vi "Main.vi"() -> ()   [LabVIEW 2018]
uses:
  Banda--control.ctl
  Banda Tolerancia--control.ctl
  states--control.ctl
  data--control.ctl
panel:
  out "in E12?":bool caption="Cumple E12?"
  out "in E24?":bool caption="Cumple E24?"
  in  "Tol":T1 caption="Tolerancia"
  out "Tol":u32(colorbox)
  out "3b":u32(colorbox)
  out "2b":u32(colorbox)
  out "1b":u32(colorbox)
  in  "stop":bool
  in  "3° banda":T2
  in  "2° banda":T2
  in  "1° banda":T2
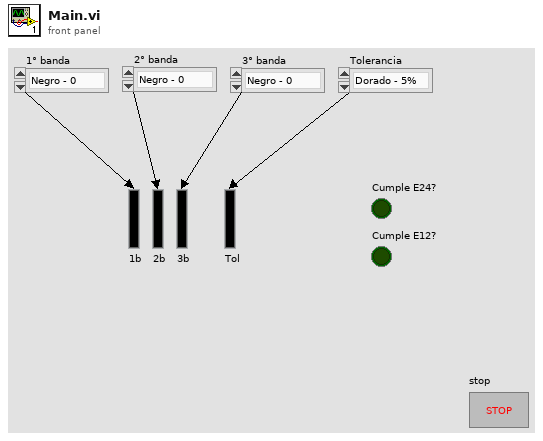
[diagram p1: front panel]
types:
  T1 = typedef "Banda Tolerancia--control.ctl" = enum16{"Dorado - 5%", "Plata - 10%"}
  T2 = typedef "Banda--control.ctl" = enum16{"Negro - 0", "Marrón - 1", "Rojo - 2", "Naranja - 3", "Amarillo - 4", "Verde - 5", "Azul - 6", "Violeta - 7", "Gris - 8", "Blanco - 9"}
  T3 = typedef "data--control.ctl" = cluster{"Number":i32, "Sting":string, "Boolean":bool, "1b Refn":refnum<vi>, "2b Refn":refnum<vi>, "3b Refn":refnum<vi>, "Tol Refn":refnum<vi>, "E24 Series":u8[], "E12 Series":u8[], "in E24?":bool, "in E12?":bool, "1° banda":T2, "2° banda":T2, "3° banda":T2, "Tolerancia":T1, "band 1":u32, "band 2":u32, "band 3":u32, "Tol":u32}
  T4 = typedef "states--control.ctl" = enum16{"Initialize", "Read E24 Series", "Read E12 Series", "Initialize Colors", "Wait", "Set Resistance Colors", "Verify E12 Series", "Verify E24 Series ", "Set Tol", "Error", "Shutdown"}
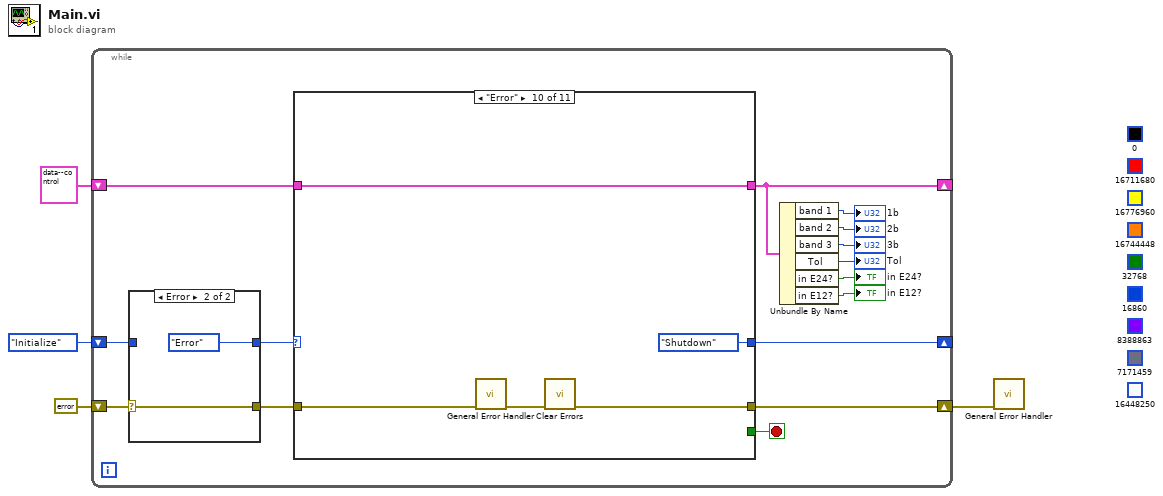
[diagram p0: block diagram]
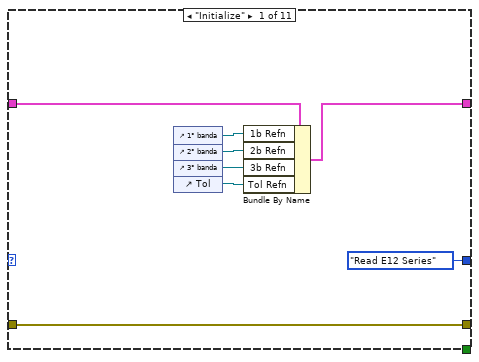
[diagram p3: hidden frame]
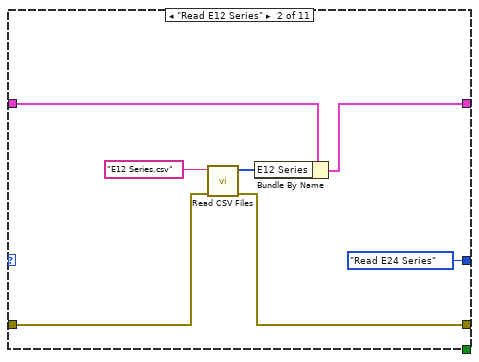
[diagram p4: hidden frame]
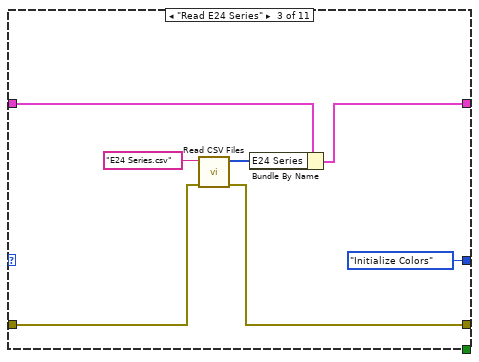
[diagram p5: hidden frame]
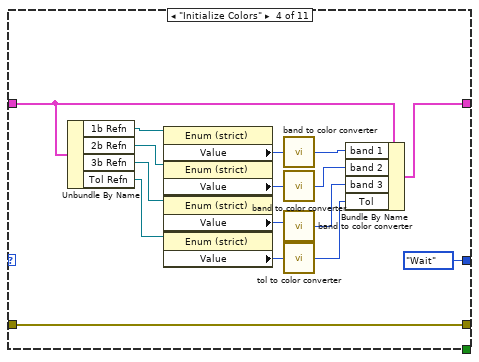
[diagram p6: hidden frame]
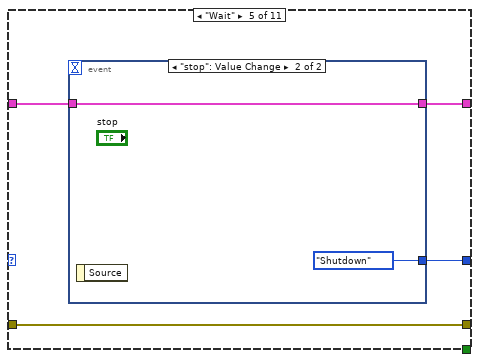
[diagram p7: hidden frame]
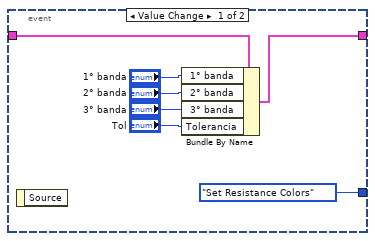
[diagram p8: hidden frame]
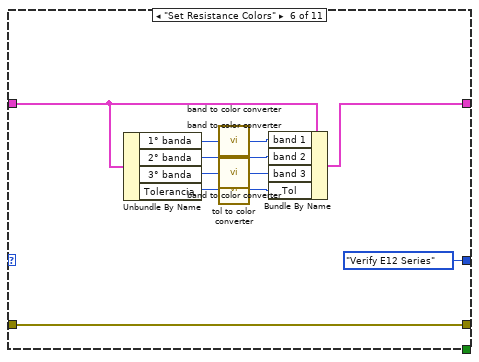
[diagram p9: hidden frame]
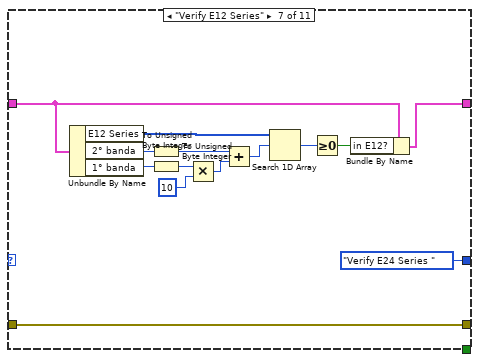
[diagram p10: hidden frame]
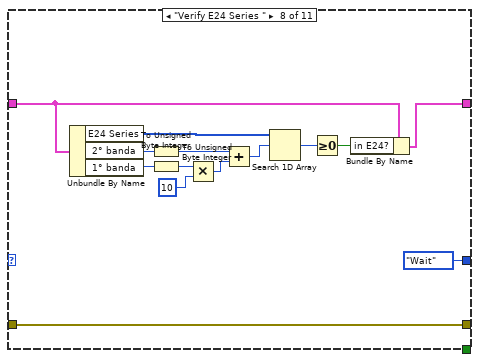
[diagram p11: hidden frame]
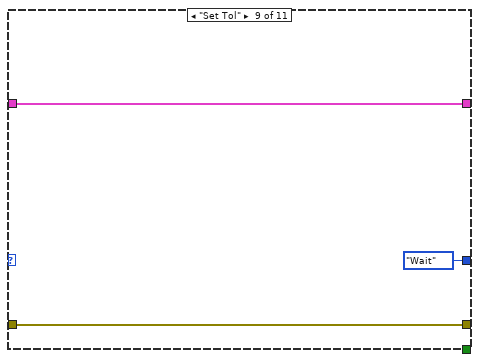
[diagram p12: hidden frame]
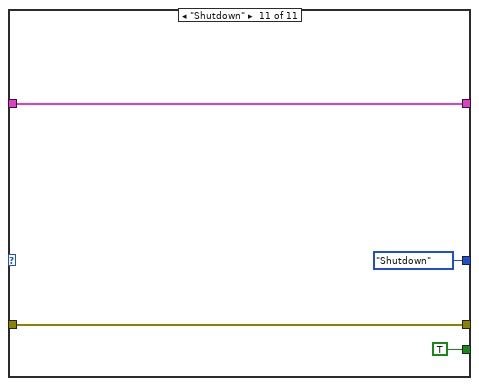
[diagram p13: hidden frame]
diagram:
  (unwired) u32 16448250
  (unwired) u32 7171459
  (unwired) u32 8388863
  (unwired) u32 16860
  (unwired) u32 32768
  (unwired) u32 16744448
  (unwired) u32 16776960
  (unwired) u32 16711680
  (unwired) u32 0
  n1 = while {
    shift-right: [w13] -> _
    shift-left: states--control."Initialize" -> [w19]
    shift-right: [w15] -> w1
    shift-left: errorcluster {"status"=FALSE, "code"=0, "source"=""} ("error constant") -> [w18]
    shift-right: [w11] -> _
    shift-left: T3 {"Number"=0, "Sting"="", "Boolean"=FALSE, "1b Refn"=refnum, "2b Refn"=refnum, "3b Refn"=refnum, "Tol Refn"=refnum, "E24 Series"=[], "E12 Series"=[], "in E24?"=FALSE, "in E12?"=FALSE, "1° banda"=enum."Negro - 0", "2° banda"=enum."Negro - 0", "3° banda"=enum."Negro - 0", "Tolerancia"=enum."Dorado - 5%", "band 1"=0, "band 2"=0, "band 3"=0, "Tol"=0} -> [w14]
    stop <- w12 stop-if-true
    n2 = case shown="Error" w18 {
      selector: w18 -> [w20 w23]
      tunnel: w19 -> [w21 _]
      tunnel: [w21 states--control."Error"] -> w17
      tunnel: [w20 w23] -> w16
      frame No Error {
      }
      frame Error {
      }
    }
    n3 = case shown="\"Error\"" w17 {
      tunnel: w16 -> [w28 w35 w43 w61 w65 w83 w100 w114 w117 w119 w126]
      tunnel: [w28 w34 w42 w61 w65 w83 w100 w114 w117 w120 w126] -> w15
      tunnel: w14 -> [w30 w38 w41 w50 w64 w80 w88 w102 w115 w122 w125]
      tunnel: [w29 w37 w40 w53 w63 w79 w87 w101 w115 w122 w125] -> w11
      tunnel: [states--control."Read E12 Series" states--control."Read E24 Series" states--control."Initialize Colors" states--control."Wait" w62 states--control."Verify E12 Series" states--control."Verify E24 Series " states--control."Wait" states--control."Wait" states--control."Shutdown" states--control."Shutdown"] -> w13
      tunnel: [_ _ _ _ _ _ _ _ _ _ TRUE] -> w12
      frame "Initialize" {
        n4 = control-ref of="1° banda"() -> (w27:refnum<vi>)
        n5 = control-ref of="2° banda"() -> (w26:refnum<vi>)
        n6 = control-ref of="3° banda"() -> (w25:refnum<vi>)
        n7 = control-ref of="Tol"() -> (w24:refnum<vi>)
        n8 = Bundle By Name(cluster=w30, "1b Refn"=w27, "2b Refn"=w26, "3b Refn"=w25, "Tol Refn"=w24) -> (w29:T3)
      }
      frame "Read E12 Series" {
        n9 = call "Read CSV Files.vi"("error in (no error)"=w35, "String"="E12 Series.csv") -> ("error out"=w34:errorcluster, "Series"=w33:u8[])  [unwired: 8 in]
        n10 = Bundle By Name(cluster=w38, "E12 Series"=w33) -> (w37:T3)
      }
      frame "Read E24 Series" {
        n11 = call "Read CSV Files.vi"("error in (no error)"=w43, "String"="E24 Series.csv") -> ("error out"=w42:errorcluster, "Series"=w44:u8[])  [unwired: 8 in]
        n12 = Bundle By Name(cluster=w41, "E24 Series"=w44) -> (w40:T3)
      }
      frame "Initialize Colors" {
        n13 = Unbundle By Name(w50) -> ("1b Refn"=w49:refnum<vi>, "2b Refn"=w48:refnum<vi>, "3b Refn"=w47:refnum<vi>, "Tol Refn"=w46:refnum<vi>)
        n14 = property class="Enum (strict)"(reference=w49) -> ("Value"=w60:T2)  [unwired: 1 in, 2 out]
        n15 = property class="Enum (strict)"(reference=w48) -> ("Value"=w59:T2)  [unwired: 1 in, 2 out]
        n16 = property class="Enum (strict)"(reference=w47) -> ("Value"=w52:T2)  [unwired: 1 in, 2 out]
        n17 = property class="Enum (strict)"(reference=w46) -> ("Value"=w58:T1)  [unwired: 1 in, 2 out]
        n18 = call "band to color converter.vi"("Banda"=w60) -> ("Color"=w57:u32)  [unwired: 6 in]
        n19 = call "band to color converter.vi"("Banda"=w59) -> ("Color"=w56:u32)  [unwired: 6 in]
        n20 = call "band to color converter.vi"("Banda"=w52) -> ("Color"=w55:u32)  [unwired: 6 in]
        n21 = call "tol to color converter.vi"("Tolerancia"=w58) -> ("Color"=w54:u32)  [unwired: 6 in]
        n22 = Bundle By Name(cluster=w50, "band 1"=w57, "band 2"=w56, "band 3"=w55, "Tol"=w54) -> (w53:T3)
      }
      frame "Wait" {
        n23 = event shown="[1] \"stop\": Value Change" {
          selector: _ -> [_ _]
          dyn-events: _ -> [_ _]
          timeout: _ -> [_ _]
          tunnel: w64 -> [w72 w74]
          tunnel: [w71 w74] -> w63
          tunnel: [states--control."Set Resistance Colors" states--control."Shutdown"] -> w62
          event Value Change {
            n24 = event-data() -> ()  [unwired: 1 in, 1 out]
            n25 = Bundle By Name(cluster=w72, "1° banda"="1° banda", "2° banda"="2° banda", "3° banda"="3° banda", "Tolerancia"="Tol") -> (w71:T3)
          }
          event "stop": Value Change {
            n26 = event-data() -> ()  [unwired: 1 in, 1 out]
          }
        }
      }
      frame "Set Resistance Colors" {
        n27 = Unbundle By Name(w80) -> ("1° banda"=w85:T2, "2° banda"=w82:T2, "3° banda"=w84:T2, "Tolerancia"=w81:T1)
        n28 = call "band to color converter.vi"("Banda"=w85) -> ("Color"=w78:u32)  [unwired: 6 in]
        n29 = call "band to color converter.vi"("Banda"=w82) -> ("Color"=w77:u32)  [unwired: 6 in]
        n30 = call "band to color converter.vi"("Banda"=w84) -> ("Color"=w76:u32)  [unwired: 6 in]
        n31 = call "tol to color converter.vi"("Tolerancia"=w81) -> ("Color"=w75:u32)  [unwired: 6 in]
        n32 = Bundle By Name(cluster=w80, "band 1"=w78, "band 2"=w77, "band 3"=w76, "Tol"=w75) -> (w79:T3)
      }
      frame "Verify E12 Series" {
        n33 = Unbundle By Name(w88) -> ("E12 Series"=w92:u8[], "2° banda"=w98:T2, "1° banda"=w97:T2)
        n34 = To Unsigned Byte Integer(number=w98) -> (unsigned 8bit integer=w94:u8)
        n35 = To Unsigned Byte Integer(number=w97) -> (unsigned 8bit integer=w96:u8)
        n36 = Multiply(x=w96, y=u8 10) -> (x*y=w93:u8)
        n37 = Add(x=w94, y=w93) -> (x+y=w91:u8)
        n38 = Search 1D Array(1D array=w92, element=w91) -> (index of element=w90:i32)  [unwired: 1 in]
        n39 = Greater Or Equal To 0?(x=w90) -> (x >= 0?=w89:bool)
        n40 = Bundle By Name(cluster=w88, "in E12?"=w89) -> (w87:T3)
      }
      frame "Verify E24 Series " {
        n41 = Unbundle By Name(w102) -> ("E24 Series"=w106:u8[], "2° banda"=w112:T2, "1° banda"=w111:T2)
        n42 = To Unsigned Byte Integer(number=w112) -> (unsigned 8bit integer=w108:u8)
        n43 = To Unsigned Byte Integer(number=w111) -> (unsigned 8bit integer=w110:u8)
        n44 = Multiply(x=w110, y=u8 10) -> (x*y=w107:u8)
        n45 = Add(x=w108, y=w107) -> (x+y=w105:u8)
        n46 = Search 1D Array(1D array=w106, element=w105) -> (index of element=w104:i32)  [unwired: 1 in]
        n47 = Greater Or Equal To 0?(x=w104) -> (x >= 0?=w103:bool)
        n48 = Bundle By Name(cluster=w102, "in E24?"=w103) -> (w101:T3)
      }
      frame "Set Tol" {
      }
      frame "Error" {
        n49 = call <vilib>:"General Error Handler.vi"("error in (no error)"=w119) -> ("error out"=w118:errorcluster)  [unwired: 10 in, 4 out]
        n50 = call <vilib>:"Clear Errors.vi"("error in (no error)"=w118) -> ("error out"=w120:errorcluster)  [unwired: 5 in, 1 out]
      }
      frame "Shutdown" {
      }
    }
    n51 = Unbundle By Name(w11) -> ("band 1"=→"1b":u32, "band 2"=→"2b":u32, "band 3"=→"3b":u32, "Tol"=→"Tol":u32, "in E24?"=→"in E24?":bool, "in E12?"=→"in E12?":bool)
  }
  n52 = call <vilib>:"General Error Handler.vi"("error in (no error)"=w1) -> ()  [unwired: 10 in, 5 out]
